vi "ALTS-2015 LV2GBL User Info.vi"(7 "Options":enum16{"Read all", "Write all"}(ring), 8 "error in":errorcluster, 11 "User Info":T1) -> (0 "error out":errorcluster, 3 "User Info Out":T1)   [LabVIEW 2013]
uses:
  Controls/ALTS-2015 User Info Cluster.ctl
panel:
  in  "User":string
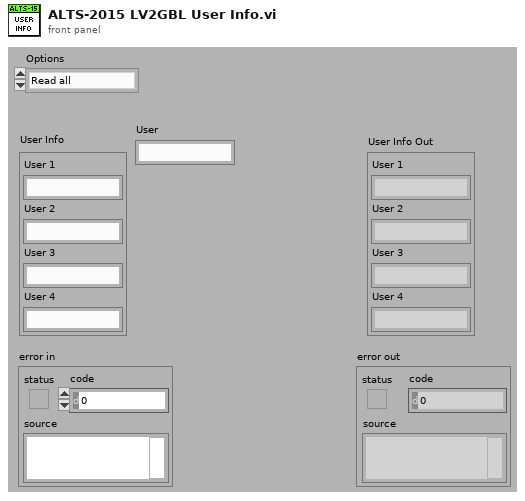
[diagram p1: front panel]
types:
  T1 = typedef "ALTS-2015 User Info Cluster.ctl" = cluster{"User 1":string, "User 2":string, "User 3":string, "User 4":string}
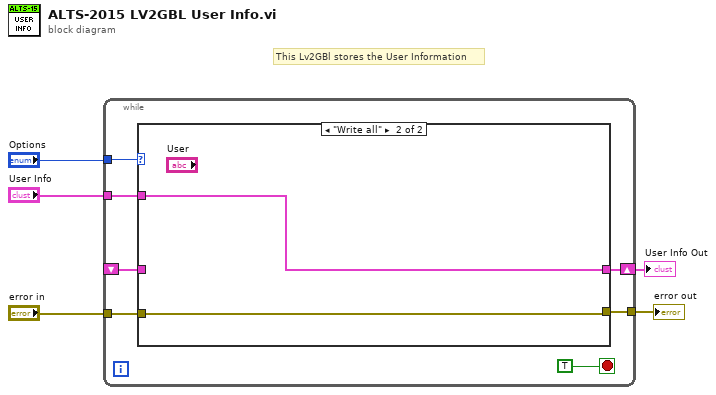
[diagram p0: block diagram]
diagram:
  # "This Lv2GBl stores the User Information"
  n1 = while {
    shift-right: [w10] -> w1
    shift-left: _ -> [w11]
    tunnel: "Options" -> [w9]
    tunnel: "User Info" -> [w8]
    tunnel: "error in" -> [w7]
    tunnel: [w6] -> w2
    stop <- TRUE stop-if-true
    n2 = case shown="\"Write all\"" w9 {
      tunnel: w11 -> [w14 _]
      tunnel: [w14 w16] -> w10
      tunnel: w8 -> [_ w16]
      tunnel: [w13 w15] -> w6
      tunnel: w7 -> [w13 w15]
      frame "Read all", Default {
      }
      frame "Write all" {
      }
    }
  }
  "error out" <- w2
  "User Info Out" <- w1
